vi "svl_Channel Info Units.vi"(6 "include weighting if dB On FALSE":bool=TRUE, 8 "error in (no error)":errorcluster, 9 "linear/dB":enum16{"linear", "dB"}(ring), 10 "channel info":T1={"sensor sensitivity"=1000.0, "engineering units"=1, "dB reference"=1.0, "custom label"="EU", "weighting filter"=0, "pregain"=0.0} {"pregain" format="%.2f"; "weighting filter" items=["Linear", "A-weighting", "B-weighting", "C-weighting", "ITU-R 468-4", "Dolby", "CCITT", "C-message", "Wb", "Wc", "Wd", "We", "Wf", "Wh", "Wj", "Wk", "Wm", "AES17 20 kHz lowpass", "AES17 40 kHz lowpass", "AES17 20 kHz highpass", "AES17 40 kHz highpass"]; "dB reference" format="%^.1e"; "engineering units" items=["custom..."=0, "V"=1, "A"=21, "C"=30, "pC"=31, "s"=32, "-"=29, "Pa"=2, "N"=20, "g"=3, "m/s^2"=4, "m/s"=5, "m"=6, "mm/s"=12, "mm"=13, "micron/s"=14, "micron"=15, "in/s^2"=7, "in/s"=8, "in"=9, "mil/s"=10, "mil"=11, "rad/s^2"=16, "rad/s"=17, "rad"=18, "deg/s^2"=26, "deg/s"=27, "deg"=28, "RPM"=22, "cycle/s^2"=23, "Hz"=24, "cycle"=25, "strain"=19]; "sensor sensitivity" format="%#_5f"}) -> (0 "error out":errorcluster, 3 "unit label":string)   [LabVIEW 2017]
uses:
  <vilib>/addons/_NISVFA/_Shared subVIs/Controls/svc_Channel Info.ctl
  <vilib>/addons/_NISVFA/_Shared subVIs/Controls/svc_Engineering Units Text Ring.ctl
  <vilib>/addons/_NISVFA/_Shared subVIs/Controls/svc_Weighting Filter Text Ring.ctl
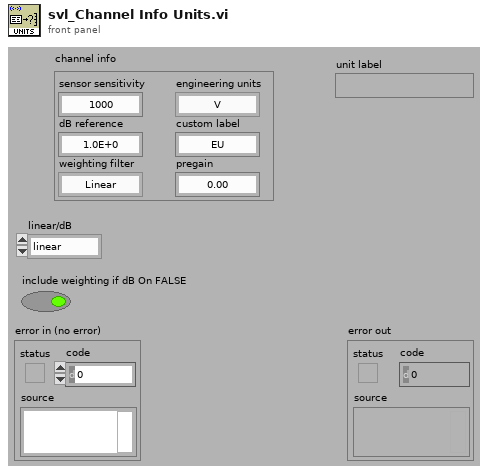
[diagram p1: front panel]
types:
  T1 = typedef "svc_Channel Info.ctl" = cluster{"sensor sensitivity":dbl, "engineering units":T2, "dB reference":dbl, "custom label":string, "weighting filter":T3, "pregain":dbl}
  T2 = typedef "svc_Engineering Units Text Ring.ctl" = u16
  T3 = typedef "svc_Weighting Filter Text Ring.ctl" = u16
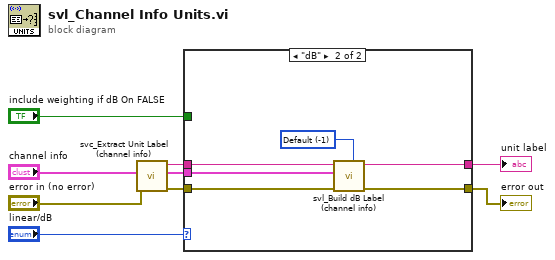
[diagram p0: block diagram]
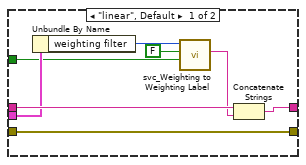
[diagram p2: hidden frame]
diagram:
  n1 = call <vilib>:"svc_Extract Unit Label (channel info).vi"("error in (no error)"="error in (no error)", "channel info"="channel info") -> ("error out"=w3:errorcluster, "channel info"=w5:T1, "unit label"=w4:string)  [unwired: 7 in]
  n2 = case shown="\"dB\"" "linear/dB" {
    tunnel: "include weighting if dB On FALSE" -> [w11 _]
    tunnel: w5 -> [w15 w23]
    tunnel: w3 -> [w17 w22]
    tunnel: w4 -> [w16 w21]
    tunnel: [w14 w20] -> w1
    tunnel: [w17 w19] -> w2
    frame "linear", Default {
      n3 = Unbundle By Name(w15) -> ("weighting filter"=w13:T3)
      n4 = call <vilib>:"svc_Weighting to Weighting Label.vi"("include weighting if dB On False (T)"=w11, "dB On (T)"=FALSE, "weighting filter"=w13) -> ("weighting string"=w10:string)  [unwired: 7 in, 1 out]
      n5 = Concatenate Strings(w16, w10) -> (w14:string)
    }
    frame "dB" {
      w18 = i16 -1 items=["Default"=-1, "Engineering"=0, "Exponential"=1, "Fractional"=2] ("number format")
      n6 = call <vilib>:"svl_Build dB Label (channel info).vi"("number format"=w18, "error in (no error)"=w22, "channel info"=w23, "EU label"=w21) -> ("error out"=w19:errorcluster, "dB label"=w20:string)  [unwired: 4 in, 2 out]
    }
  }
  "error out" <- w2
  "unit label" <- w1
